vi "UTL_ConnectCtrls.vi"(8 "error in (no error)":errorcluster, 11 "Array CtrlCluster":T1(array[cluster])) -> (0 "error out":errorcluster)   [LabVIEW 2019]
uses:
  Variable global de carga.vi
  <vilib>/Plasmionique/MB Master/MB_Master_Serial/MB_Master_Serial.lvclass
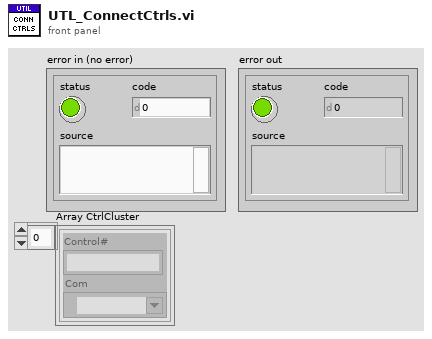
[diagram p1: front panel]
types:
  T1 = cluster{"Control#":string, "Com":refnum<visa-resource-name>}[]
  T2 = cluster{"baud rate (bps)":u32, "stop bits":u16, "parity":u16, "flow control":u16, "timeout":u32, "retries":i32}
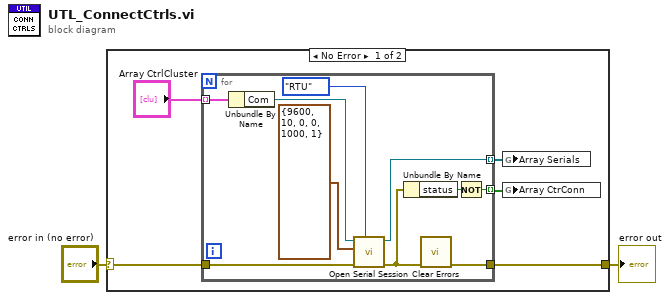
[diagram p0: block diagram]
diagram:
  n1 = case shown="No Error" "error in (no error)" {
    selector: "error in (no error)" -> [w5 w18]
    tunnel: [w4 w18] -> w1
    frame No Error {
      n2 = for {
        tunnel: [w8] -> w4
        tunnel: w5 -> [w15]
        tunnel: [w14] -> w7 mode=indexing
        tunnel: "Array CtrlCluster" -> [w13] mode=indexing
        tunnel: [w11] -> w6 mode=indexing
        n3 = Unbundle By Name(w13) -> ("Com"=w12:refnum<visa-resource-name>)
        n4 = call <vilib>:"Open Serial Session.vi"("Mode (RTU)"=enum16{"RTU", "ASCII"}."RTU", "Error in"=w15, "Serial Config"=T2 {"baud rate (bps)"=9600, "stop bits"=10, "parity"=0, "flow control"=0, "timeout"=1000, "retries"=1}, "VISA Resource"=w12) -> ("Error out"=w9:errorcluster, "MB_Serial session"=w14:refnum<class "MB_Master_Serial.lvclass">)  [unwired: 6 in]
        n5 = Unbundle By Name(w9) -> ("status"=w10:bool)
        n6 = call <vilib>:"Clear Errors.vi"("error in (no error)"=w9) -> ("error out"=w8:errorcluster)  [unwired: 5 in, 1 out]
        n7 = Not(x=w10) -> (.not. x?=w11:bool)
      }
      n8 = global write "Variable global de carga.vi" "Array Serials"(w7) -> ()
      n9 = global write "Variable global de carga.vi" "Array CtrConn"(w6) -> ()
    }
    frame Error {
    }
  }
  "error out" <- w1
